vi "Open.vi"(4 "Gyro Full Scale Range":T7, 6 "Accel Full Scale Range":T8, 7 "I2C Channel":u8, 8 "Error In":errorcluster, 9 "Clock Source":u8=1, 10 "Device Address":T9=enum."0x69", 11 "LINX Resource":T1) -> (0 "Error Out":errorcluster, 3 "LINX Resource":T1)   [LabVIEW 2011, in "LVH-LINX.lvlib" / "MPU60X0.lvlib"]
doc: "Initializes the MPU-60X0 device setting the clock source and the full ranges for the accelerometer and gyro.\n\nOriginal Code Contributed By NathanB"
uses:
  MPU60X0.lvlib
  DeviceAddresses.ctl
  AccelFullScaleRanges.ctl
  GyroFullScaleRanges.ctl
  Private/Type Defs/LINX Ref.ctl
  Private/Type Defs/Platform.ctl
  Private/Type Defs/Interface.ctl
  Private/Device/Type Defs/LINX Device Config.ctl
  Private/Device/Type Defs/TCP Config.ctl
  Private/Device/Type Defs/Channels.ctl
  LVH-LINX.lvlib
  Private/Device/Device.lvlib
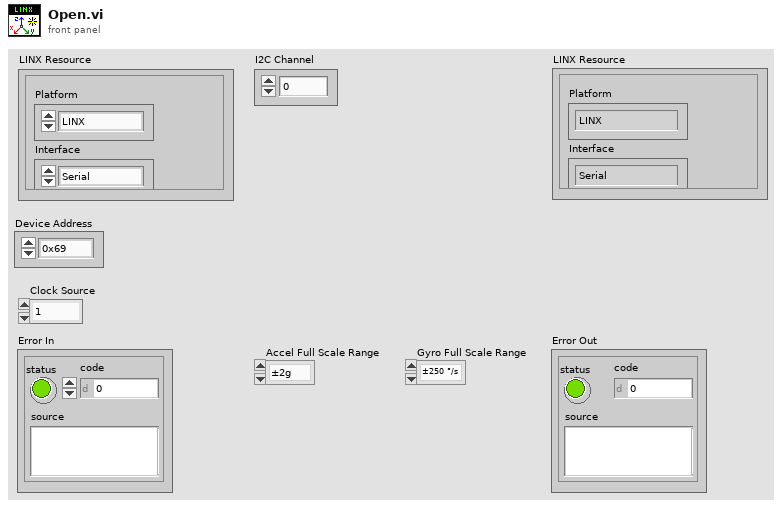
[diagram p1: front panel]
types:
  T1 = typedef "LVH-LINX.lvlib/LINX Ref.ctl" = cluster{"Platform":T2, "Interface":T3, "LINX Device Config":T4}
  T2 = typedef "LVH-LINX.lvlib/Platform.ctl" = enum16{"LINX", "myRIO"}
  T3 = typedef "LVH-LINX.lvlib/Interface.ctl" = enum16{"Serial", "TCP"}
  T4 = typedef "LVH-LINX.lvlib/Device.lvlib/LINX Device Config.ctl" = cluster{"Interface":T3, "COM Port":refnum<visa-resource-name>, "TCP Configuration":T5, "Device Family":u8, "Device ID":u8, "Device Name":string, "TCP Ref":refnum<k5>, "Channels":T6}
  T5 = typedef "LVH-LINX.lvlib/Device.lvlib/TCP Config.ctl" = cluster{"IP Address":string, "Port":u16}
  T6 = typedef "LVH-LINX.lvlib/Channels.ctl" = cluster{"DI":u8[], "DO":u8[], "AI":u8[], "AO":u8[], "PWM":u8[], "QE":u8[], "UART":u8[], "I2C 2":u8[], "SPI":u8[], "CAN":u8[], "Servo":u8[], "AI Ref (V)":dbl, "AO Ref (V)":dbl, "AO Resolution (Bits)":u8}
  T7 = typedef "LVH-LINX.lvlib/MPU60X0.lvlib/GyroFullScaleRanges.ctl" = enum8{"±250 °/s", "±500 °/s", "±1000 °/s", "±2000 °/s"}
  T8 = typedef "LVH-LINX.lvlib/MPU60X0.lvlib/AccelFullScaleRanges.ctl" = enum16{"±2g", "±4g", "±8g", "±16g"}
  T9 = typedef "LVH-LINX.lvlib/MPU60X0.lvlib/DeviceAddresses.ctl" = enum16{"0x68", "0x69"}
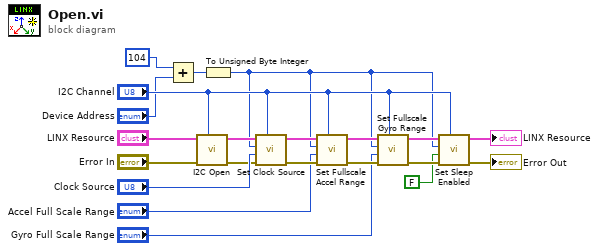
[diagram p0: block diagram]
diagram:
  n1 = Add(x=u8 104 ("Clock Source"), y="Device Address") -> (x+y=w2:u16)
  n2 = call "I2C Open.vi"("I2C Channel (0)"="I2C Channel", "Error In"="Error In", "LINX Resource"="LINX Resource") -> ("Error Out"=w6:errorcluster, "LINX Resource"=w8:T1)  [unwired: 7 in]
  n3 = To Unsigned Byte Integer(number=w2) -> (unsigned 8bit integer=w1:u8)
  n4 = call "Set Clock Source.vi"("I2C Channel"="I2C Channel", "Error In"=w6, "Clock Source"="Clock Source", "Device Address"=w1, "LINX Resource"=w8) -> ("Error Out"=w19:errorcluster, "LINX Resource"=w12:T1)  [unwired: 5 in]
  n5 = call "Set Fullscale Accel Range.vi"("I2C Channel"="I2C Channel", "Error In"=w19, "Accel Full Scale Range"="Accel Full Scale Range", "Device Address"=w1, "LINX Resource"=w12) -> ("Error Out"=w18:errorcluster, "LINX Resource"=w11:T1)  [unwired: 5 in]
  n6 = call "Set Fullscale Gyro Range.vi"("I2C Channel"="I2C Channel", "Error In"=w18, "Gyro Full Scale Range"="Gyro Full Scale Range", "Device Address"=w1, "LINX Resource"=w11) -> ("Error Out"=w17:errorcluster, "LINX Resource"=w21:T1)  [unwired: 5 in]
  n7 = call "Set Sleep Enabled.vi"("I2C Channel"="I2C Channel", "Error In"=w17, "Sleep?"=FALSE, "Device Address"=w1, "LINX Resource"=w21) -> ("Error Out"=→"Error Out":errorcluster, "LINX Resource"=→"LINX Resource":T1)  [unwired: 5 in]
